vi "시작 글로벌.vi"() -> ()   [LabVIEW 2017]
panel:
  out "자동시작 불리언":bool
  out "수동시작 불리언":bool
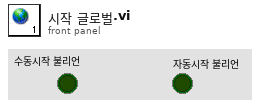
[diagram p1: front panel]
diagram:
